vi "Pneumatic Controller.vi"(8 "State In":T1, 9 "Time Limit Down":i32=1000, 10 "Time Limit Up":i32=1000, 11 "Notifier in":refnum<notifier>) -> (2 "State Out":T1, 3 "Value":T2)   [LabVIEW 2015]
uses:
  Pneumatic State Machine.ctl
  <vilib>/Rock Robotics/WPI/Solenoid/WPI_SolenoidValue.ctl
  Pneumatic Commands.ctl
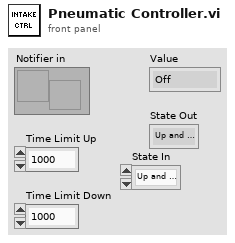
[diagram p1: front panel]
types:
  T1 = typedef "Pneumatic State Machine.ctl" = enum16{"Up and Pressure", "Down and Pressue", "Up and Float", "Down and Float"}
  T2 = typedef "WPI_SolenoidValue.ctl" = enum16{"Off", "On", "Forward", "Reverse"}
  T3 = typedef "Pneumatic Commands.ctl" = enum16{"Go Up", "Go Down", "Nothing"}
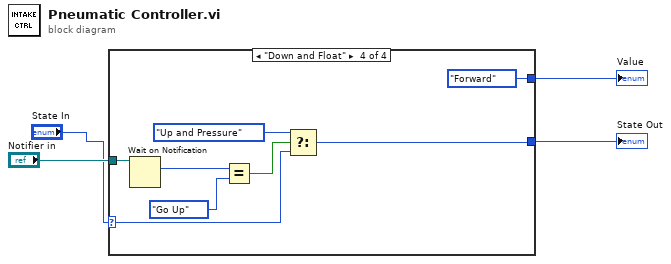
[diagram p0: block diagram]
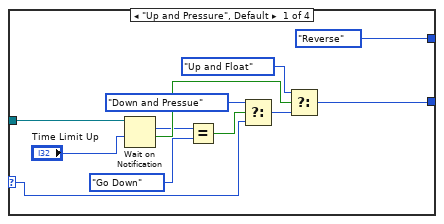
[diagram p2: hidden frame]
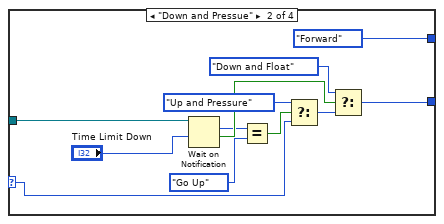
[diagram p3: hidden frame]
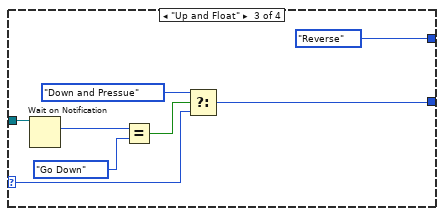
[diagram p4: hidden frame]
diagram:
  n1 = case shown="\"Down and Float\"" "State In" {
    selector: "State In" -> [w7 w18 w32 w40]
    tunnel: [WPI_SolenoidValue."Reverse" ("Value") WPI_SolenoidValue."Forward" ("Value") WPI_SolenoidValue."Reverse" ("Value") WPI_SolenoidValue."Forward" ("Value")] -> w3
    tunnel: [w5 w17 w35 w43] -> w4
    tunnel: "Notifier in" -> [w9 w23 w30 w38]
    frame "Up and Pressure", Default {
      n2 = Wait on Notification(notifier=w9, timeout in ms (-1)="Time Limit Up") -> (notification=w8:T3, timed out?=w10:bool)  [unwired: 2 in, 2 out]
      n3 = Equal?(x=w8, y=Pneumatic_Commands."Go Down") -> (x = y?=w12:bool)
      n4 = Select(t=Pneumatic_State_Machine."Down and Pressue", s=w12, f=w7) -> (s? t:f=w6:T1)
      n5 = Select(t=Pneumatic_State_Machine."Up and Float", s=w10, f=w6) -> (s? t:f=w5:T1)
    }
    frame "Down and Pressue" {
      n6 = Wait on Notification(notifier=w23, timeout in ms (-1)="Time Limit Down") -> (notification=w20:T3, timed out?=w21:bool)  [unwired: 2 in, 2 out]
      n7 = Equal?(x=w20, y=Pneumatic_Commands."Go Up") -> (x = y?=w24:bool)
      n8 = Select(t=Pneumatic_State_Machine."Up and Pressure", s=w24, f=w18) -> (s? t:f=w19:T1)
      n9 = Select(t=Pneumatic_State_Machine."Down and Float", s=w21, f=w19) -> (s? t:f=w17:T1)
    }
    frame "Up and Float" {
      n10 = Wait on Notification(notifier=w30) -> (notification=w29:T3)  [unwired: 3 in, 3 out]
      n11 = Equal?(x=w29, y=Pneumatic_Commands."Go Down") -> (x = y?=w31:bool)
      n12 = Select(t=Pneumatic_State_Machine."Down and Pressue", s=w31, f=w32) -> (s? t:f=w35:T1)
    }
    frame "Down and Float" {
      n13 = Wait on Notification(notifier=w38) -> (notification=w37:T3)  [unwired: 3 in, 3 out]
      n14 = Equal?(x=w37, y=Pneumatic_Commands."Go Up") -> (x = y?=w39:bool)
      n15 = Select(t=Pneumatic_State_Machine."Up and Pressure", s=w39, f=w40) -> (s? t:f=w43:T1)
    }
  }
  "State Out" <- w4
  "Value" <- w3
